vi "Edit Instructions.vi"(0 "Instruction File":path=path "D:/modernlab-ref-architecture/src/measurement_build_automation/_Measurement Builder/Template for Package/data/instructions", 5 "Meas Name":string, 11 "error in (no error)":errorcluster) -> (15 "error out":errorcluster)   [LabVIEW 2021, in "Measurement Builder.lvlib"]
uses:
  Measurement Builder.lvlib
  <vilib>/Utility/sysdir.llb/System Directory Type.ctl
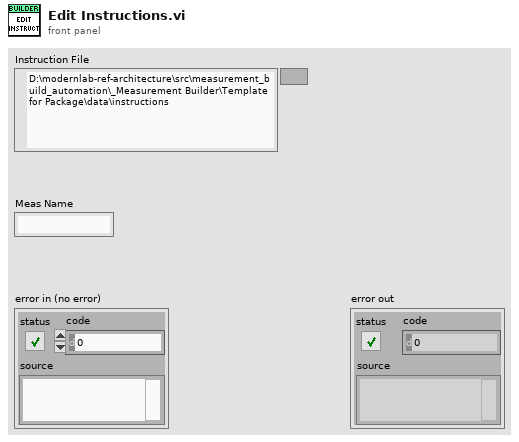
[diagram p1: front panel]
types:
  T1 = enum16{"open", "replace", "create", "open or create", "replace or create", "replace or create with confirmation"}
  T2 = typedef "System Directory Type.ctl" = i32
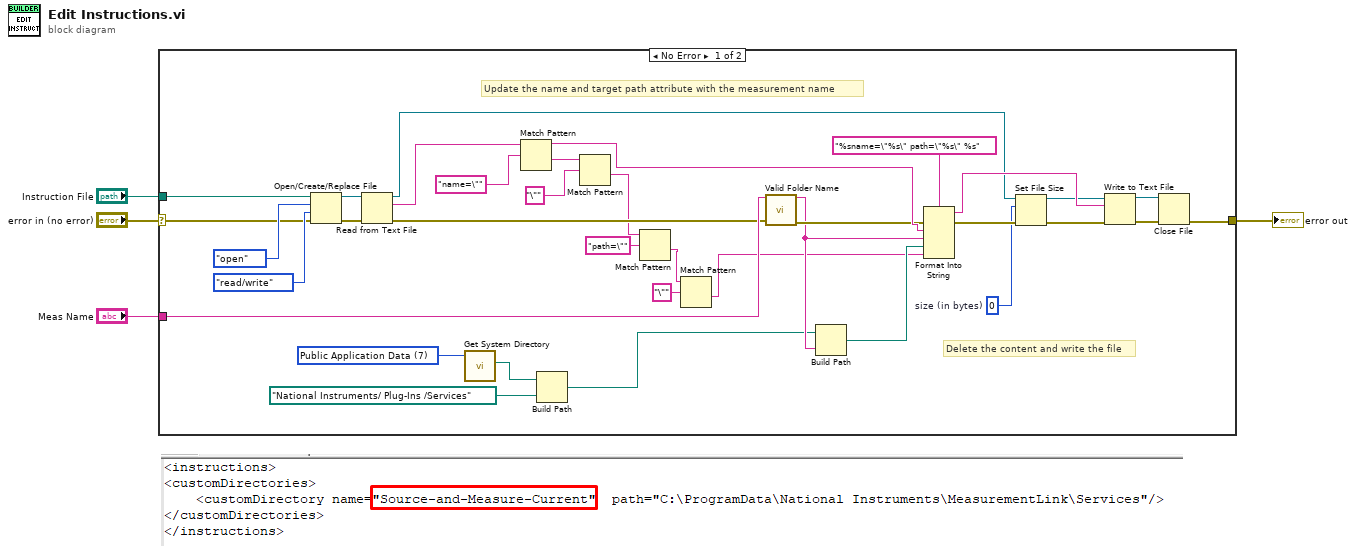
[diagram p0: block diagram]
diagram:
  n1 = case shown="No Error" "error in (no error)" {
    selector: "error in (no error)" -> [w32 w40]
    tunnel: "Instruction File" -> [w39 _]
    tunnel: [w24 w40] -> w2
    tunnel: "Meas Name" -> [w18 _]
    frame No Error {
      w8 = T2 7 items=["User Home"=0, "User Desktop"=1, "User Documents"=2, "User Application Data"=3, "User Preferences"=4, "User Temporary"=5, "Public Documents"=6, "Public Application Data"=7, "Public Preferences"=8, "Public Cache"=13, "System Core Libraries"=9, "System Installed Libraries"=10, "Application Files"=11, "Boot Volume Root"=12] ("system directory type")
      w19 = i64 0  # size (in bytes)
      # "Delete the content and write the file"
      # "Update the name and target path attribute with the measurement name"
      n2 = Open/Create/Replace File(file path (use dialog)=w39, error in=w32, operation (0:open)=T1."open", access (0:read/write)=enum16{"read/write", "read-only", "write-only"}."read/write") -> (refnum out=w36:refnum<file>, error out=w35:errorcluster)  [unwired: 2 in, 1 out]
      n3 = Read from Text File(file (use dialog)=w36, error in=w35) -> (refnum out=w21:refnum<file>, text=w34:string, error out=w17:errorcluster)  [unwired: 2 in, 1 out]
      n4 = call <vilib>:"Get System Directory.vi"("system directory type"=w8) -> ("system directory"=w7:path)  [unwired: 10 in]
      n5 = Match Pattern(string=w34, regular expression="name=\"") -> (before substring=w28:string, after substring=w31:string)  [unwired: 1 in, 2 out]
      n6 = Build Path(base path=w7, name or relative path=path "National Instruments/ Plug-Ins /Services" ("Instruction File")) -> (appended path=w6:path)
      n7 = Match Pattern(string=w31, regular expression="\"") -> (after substring=w15:string)  [unwired: 1 in, 3 out]
      n8 = Match Pattern(string=w15, regular expression="path=\"") -> (after substring=w12:string)  [unwired: 1 in, 3 out]
      n9 = Match Pattern(string=w12, regular expression="\"") -> (after substring=w9:string)  [unwired: 1 in, 3 out]
      n10 = call "Valid Folder Name.vi"("Package"=w18, "error in (no error)"=w17) -> ("Valid Package Name"=w11:string, "error out"=w16:errorcluster)  [unwired: 12 in]
      n11 = Build Path(base path=w6, name or relative path=w11) -> (appended path=w10:path)
      n12 = Format Into String(format string="%sname=\"%s\" path=\"%s\" %s", error in=w16, w28, w11, w10, w9) -> (resulting string=w27:string, error out=w23:errorcluster)  [unwired: 1 in]
      n13 = Set File Size(4:w23, 6:w19, 7:w21) -> (0:w22:errorcluster, 3:w20:refnum<file>)
      n14 = Write to Text File(file (use dialog)=w20, text=w27, error in=w22) -> (refnum out=w26:refnum<file>, error out=w25:errorcluster)  [unwired: 1 in, 1 out]
      n15 = Close File(refnum=w26, error in=w25) -> (error out=w24:errorcluster)  [unwired: 1 out]
    }
    frame Error {
    }
  }
  "error out" <- w2
